vi "RW Slave.vi"(7 "R/W Case":T2, 8 "error in (no error)":errorcluster, 10 "Async in":T1, 11 "Slave in":T3 {"FPGA"."UDVs"."To FPGA"."VS ref" format="%.0x"; "FPGA"."UDVs"."From FPGA"."VS ref" format="%.0x"; "FPGA"."VS ref" format="%.0x"; "FPGA"."Output Data"."BD Refs"."Data Reference" format="%.0x"; "FPGA"."Input Data"."BD Refs"."Data Reference" format="%.0x"; "RSI Modules"."Module Config Data"."Config Block Data Refs"."Data Reference" format="%.0x"; "RSI Modules"."CDOutput Data"."BD Refs"."Data Reference" format="%.0x"; "RSI Modules"."CDInput Data"."BD Refs"."Data Reference" format="%.0x"; "RSI Modules"."VS ref" format="%.0x"; "VS ref" format="%.0x"}) -> (0 "error out":errorcluster, 2 "Async out":T1, 3 "Slave out":T3 {"FPGA"."UDVs"."To FPGA"."VS ref" format="%.0x"; "FPGA"."UDVs"."From FPGA"."VS ref" format="%.0x"; "FPGA"."VS ref" format="%.0x"; "FPGA"."Output Data"."BD Refs"."Data Reference" format="%.0x"; "FPGA"."Input Data"."BD Refs"."Data Reference" format="%.0x"; "RSI Modules"."Module Config Data"."Config Block Data Refs"."Data Reference" format="%.0x"; "RSI Modules"."CDOutput Data"."BD Refs"."Data Reference" format="%.0x"; "RSI Modules"."CDInput Data"."BD Refs"."Data Reference" format="%.0x"; "RSI Modules"."VS ref" format="%.0x"; "VS ref" format="%.0x"})   [LabVIEW 2016, in "Scan Engine Custom Device.lvlib"]
uses:
  Scan Engine Custom Device.lvlib
  <vilib>/NI Veristand/Custom Device API/Custom Device Item Ref.ctl
  <vilib>/NI Veristand/Custom Device API/Custom Device API.lvlib
  Modules.lvlibp/RSI Module/RSI Module.lvclass
  <vilib>/NI Veristand/Custom Device API/Data Reference.ctl
  <vilib>/NI Veristand/Custom Device API/Block Data Reference.ctl
  Type Defs/Input Data.ctl
  Type Defs/Output Data.ctl
  Type Defs/RSI Module Data.ctl
  Type Defs/FPGA Data.ctl
  Type Defs/EtherCAT Slave Data.ctl
  Modules.lvlibp/RSI Module/Channel Type.ctl
  Type Defs/RW Case.ctl
  Type Defs/UDV Data Type.ctl
  Type Defs/FXP Config.ctl
  Type Defs/UDV Data.ctl
  Modules.lvlibp/RSI Module/Module Models.ctl
  Type Defs/Module Config Data.ctl
  Type Defs/Async Command.ctl
  Type Defs/Async State.ctl
  Type Defs/Async Status.ctl
  Type Defs/Async Data.ctl
  Type Defs/Mixed IO.ctl
  Type Defs/Open Module IOVs.ctl
  Type Defs/Mod Size Indexes.ctl
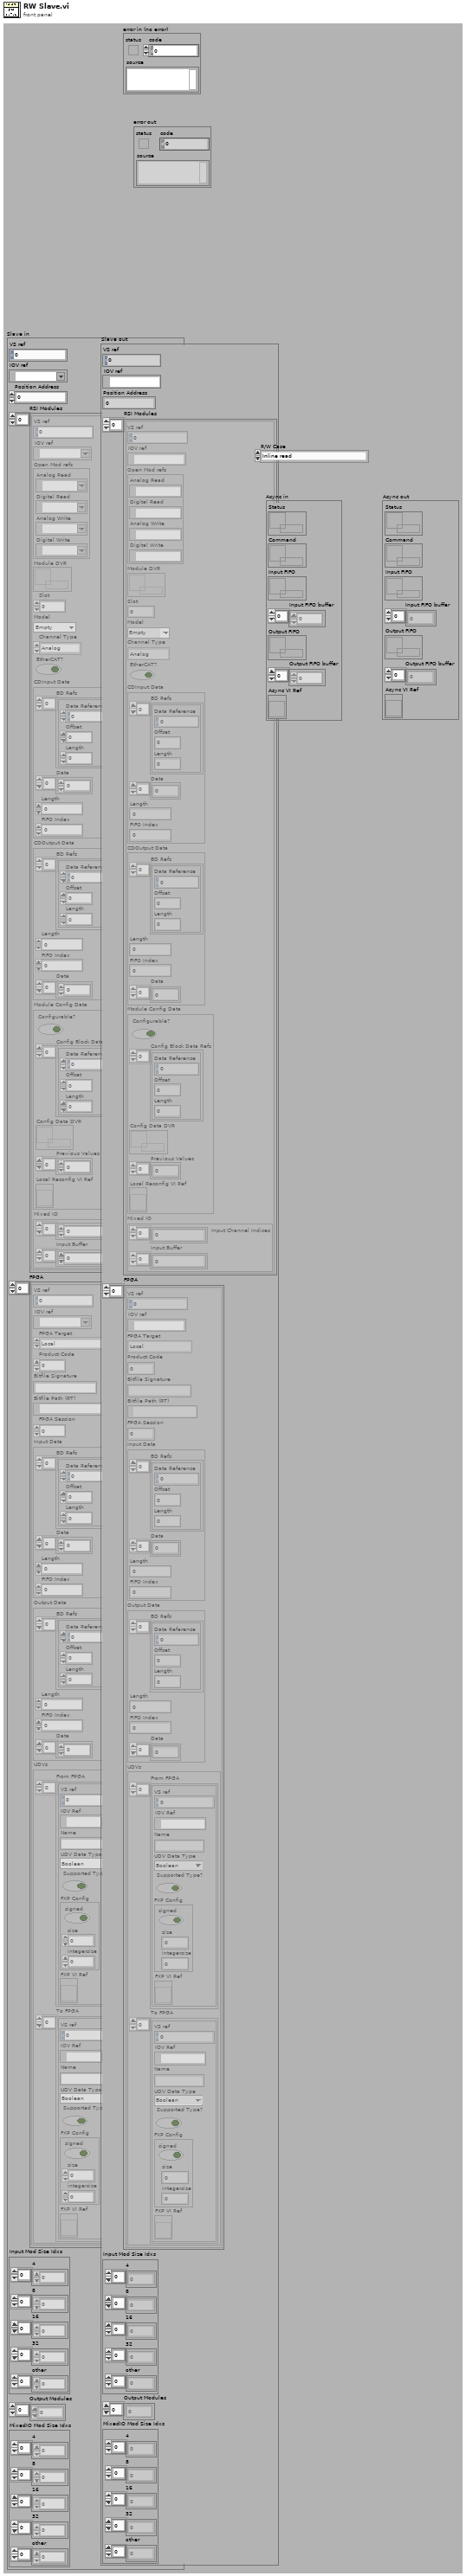
[diagram p1: front panel]
types:
  T1 = typedef "Scan Engine Custom Device.lvlib/Async Data.ctl" = cluster{"Status":refnum<queue>, "Command":refnum<queue>, "Input FIFO":refnum<k33>, "Input FIFO buffer":dbl[], "Output FIFO":refnum<k33>, "Output FIFO buffer":dbl[], "Async VI Ref":refnum<vi>}
  T2 = typedef "Scan Engine Custom Device.lvlib/RW Case.ctl" = enum16{"Inline read", "Inline write", "Async - Inline loop read", "Async - Inline loop write", "Async loop (read/write)"}
  T3 = typedef "Scan Engine Custom Device.lvlib/EtherCAT Slave Data.ctl" = cluster{"VS ref":T4, "IOV ref":refnum<k21>, "Position Address":u16, "RSI Modules":T5[], "FPGA":T15[], "Input Mod Size Idxs":T19, "Output Modules":i32[], "MixedIO Mod Size Idxs":T19}
  T4 = typedef "Custom Device API.lvlib/Custom Device Item Ref.ctl" = u64
  T5 = typedef "Scan Engine Custom Device.lvlib/RSI Module Data.ctl" = cluster{"VS ref":T4, "IOV ref":refnum<k21>, "Open Mod refs":T6, "Module DVR":refnum<data-value>, "Slot":u32, "Model":T7, "Channel Type":T8, "EtherCAT?":bool, "CDInput Data":T9, "CDOutput Data":T12, "Module Config Data":T13, "Mixed IO":T14}
  T6 = typedef "Scan Engine Custom Device.lvlib/Open Module IOVs.ctl" = cluster{"Analog Read":refnum<k21>, "Digital Read":refnum<k21>, "Analog Write":refnum<k21>, "Digital Write":refnum<k21>}
  T7 = typedef "Modules.lvlibp/RSI Module.lvclass/Module Models.ctl" = enum16{"Empty", "NI 9201", "NI 9203", "NI 9205", "NI 9206", "NI 9207", "NI 9208", "NI 9211", "NI 9213", "NI 9214", "NI 9215", "NI 9217", "NI 9219", "NI 9221", "NI 9225", "NI 9227", "NI 9229", "NI 9233", "NI 9234", "NI 9235", "NI 9236", "NI 9237", "NI 9239", "NI 9263", "NI 9264", "NI 9265", "NI 9269", "NI 9375", "NI 9401", "NI 9402", "NI 9403", "NI 9411", "NI 9421", "NI 9422", "NI 9423", "NI 9425", "NI 9426", "NI 9435", "NI 9472", "NI 9474", "NI 9475", "NI 9476", "NI 9477", "NI 9478", "NI 9481", "NI 9482", "NI 9485"}
  T8 = typedef "Modules.lvlibp/RSI Module.lvclass/Channel Type.ctl" = enum16{"Analog", "Digital"}
  T9 = typedef "Scan Engine Custom Device.lvlib/Input Data.ctl" = cluster{"BD Refs":T10[], "Data":dbl[], "Length":i32, "FIFO Index":i32}
  T10 = typedef "Custom Device API.lvlib/Block Data Reference.ctl" = cluster{"Data Reference":T11, "Offset":u64, "Length":u64}
  T11 = typedef "Custom Device API.lvlib/Data Reference.ctl" = i32
  T12 = typedef "Scan Engine Custom Device.lvlib/Output Data.ctl" = cluster{"BD Refs":T10[], "Length":i32, "FIFO Index":i32, "Data":dbl[]}
  T13 = typedef "Scan Engine Custom Device.lvlib/Module Config Data.ctl" = cluster{"Configurable?":bool, "Config Block Data Refs":T10[], "Config Data DVR":refnum<data-value>, "Previous Values":dbl[], "Local Reconfig VI Ref":refnum<vi>}
  T14 = typedef "Scan Engine Custom Device.lvlib/Mixed IO.ctl" = cluster{"Input Channel Indices":i32[], "Input Buffer":dbl[]}
  T15 = typedef "Scan Engine Custom Device.lvlib/FPGA Data.ctl" = cluster{"VS ref":T4, "IOV ref":refnum<k21>, "FPGA Target":enum16{"Local", "EtherCAT"}, "Product Code":u32, "Bitfile Signature":string, "Bitfile Path (RT)":path, "FPGA Session":u32, "Input Data":T9, "Output Data":T12, "UDVs":cluster{"From FPGA":T16[], "To FPGA":T16[]}}
  T16 = typedef "Scan Engine Custom Device.lvlib/UDV Data.ctl" = cluster{"VS ref":T4, "IOV Ref":refnum<k21>, "Name":string, "UDV Data Type":T17, "Supported Type?":bool, "FXP Config":T18, "FXP VI Ref":refnum<vi>}
  T17 = typedef "Scan Engine Custom Device.lvlib/UDV Data Type.ctl" = enum16{"Boolean", "Fixed Point", "Int8", "Int16", "Int32", "Int64", "U32 Bit Field", "UInt8", "UInt16", "UInt32", "UInt64", "Other"}
  T18 = typedef "Scan Engine Custom Device.lvlib/FXP Config.ctl" = cluster{"signed":bool, "size":u32, "integersize":i32}
  T19 = typedef "Scan Engine Custom Device.lvlib/Mod Size Indexes.ctl" = cluster{"4":i32[], "8":i32[], "16":i32[], "32":i32[], "other":i32[]}
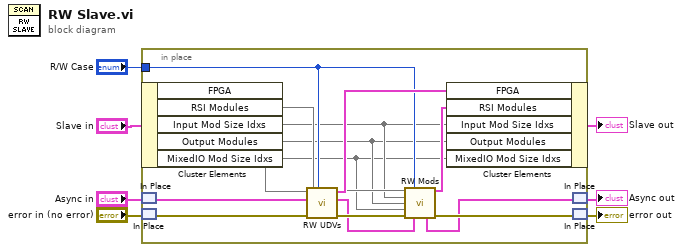
[diagram p0: block diagram]
diagram:
  n1 = in-place {
    in-place-border: "R/W Case" -> [w18]
    n2 = in-place-cluster #1("Slave in") -> ("FPGA"=w21, "RSI Modules"=w14, "Input Mod Size Idxs"=w12, "Output Modules"=w11, "MixedIO Mod Size Idxs"=w10)
    n3 = in-place-match #2("Async in") -> (w17:T1)
    n4 = in-place-match #3("error in (no error)") -> (w16:errorcluster)
    n5 = call "RW UDVs.vi"("R/W Case"=w18, "error in (no error)"=w16, "Async in"=w17, "FPGA in"=w21) -> ("error out"=w19:errorcluster, "Async out"=w9:T1, "FPGA out"=w20:T15[])  [unwired: 5 in]
    n6 = call "RW Mods.vi"("RSI Modules in"=w14, "R/W Case"=w18, "Input Mod Size Idxs"=w12, "Output modules"=w11, "MixedIO Mod Size Idxs"=w10, "error in (no error)"=w19, "Async in"=w9) -> ("RSI Modules out"=w13:T5[], "Async out"=w8:T1, "error out"=w15:errorcluster)  [unwired: 6 in]
    n7 = in-place-cluster #1("FPGA"=w20, "RSI Modules"=w13, "Input Mod Size Idxs"=w12, "Output Modules"=w11, "MixedIO Mod Size Idxs"=w10) -> (→"Slave out":cluster{})
    n8 = in-place-match #2(w8) -> (→"Async out":T1)
    n9 = in-place-match #3(w15) -> (→"error out":errorcluster)
  }
